vi "Write Timeout.vi"(8 "error in (no error)":errorcluster, 10 "Timeout":dbl, 11 "Repeat Until Timeout in":refnum<class "Repeat Until Timeout.lvclass">) -> (0 "error out":errorcluster, 3 "Repeat Until Timeout out":refnum<class "Repeat Until Timeout.lvclass">)   [LabVIEW 2021, in "BT.lvlib" / "Repeat Until Timeout.lvclass"]
uses:
  Repeat Until Timeout.lvclass
  Repeat Until Timeout.lvclass/Repeat Until Timeout.ctl
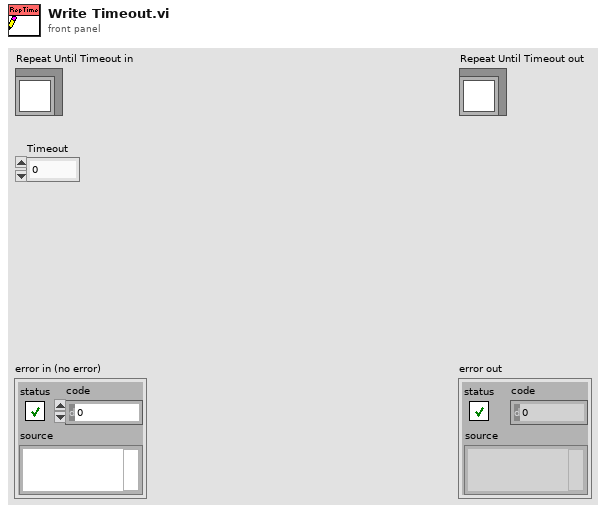
[diagram p1: front panel]
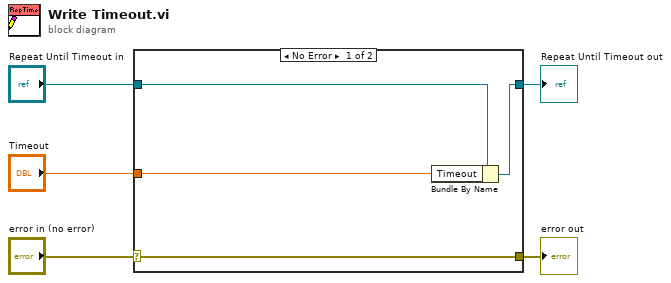
[diagram p0: block diagram]
diagram:
  n1 = case shown="No Error" "error in (no error)" {
    selector: "error in (no error)" -> [w9 w10]
    tunnel: [w9 w10] -> w4
    tunnel: [w7 w11] -> w2
    tunnel: "Repeat Until Timeout in" -> [w8 w11]
    tunnel: "Timeout" -> [w6 _]
    frame No Error {
      n2 = Bundle By Name(cluster=w8, "Timeout"=w6) -> (w7:refnum<class "Repeat Until Timeout.lvclass">)
    }
    frame Error {
    }
  }
  "error out" <- w4
  "Repeat Until Timeout out" <- w2
